vi "Set Tip String.vi"(8 "error in (no error)":errorcluster, 10 "tip string":string, 11 "ClickableText in":refnum<class "ClickableText.lvclass">) -> (0 "error out":errorcluster, 3 "ClickableText out":refnum<class "ClickableText.lvclass">)   [LabVIEW 2009, in "NavScreen.lvlib" / "ClickableText.lvclass"]
uses:
  ClickableText.lvclass
  ClickableText.lvclass/ClickableText.ctl
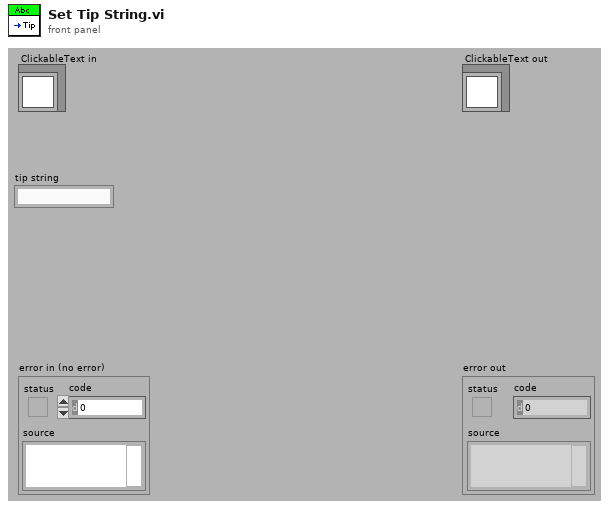
[diagram p1: front panel]
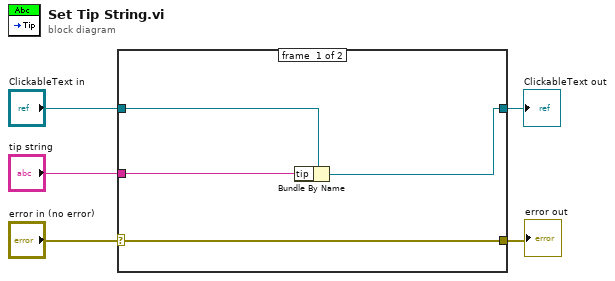
[diagram p0: block diagram]
diagram:
  n1 = case shown="No Error" "error in (no error)" {
    selector: "error in (no error)" -> [w9 w11]
    tunnel: [w9 w11] -> w4
    tunnel: [w6 w10] -> w2
    tunnel: "ClickableText in" -> [w8 w10]
    tunnel: "tip string" -> [w7 _]
    frame #0 {
      n2 = Bundle By Name(cluster=w8, "tip"=w7) -> (w6:refnum<class "ClickableText.lvclass">)
    }
    frame #1 {
    }
  }
  "error out" <- w4
  "ClickableText out" <- w2
